vi "d(f2+g2u)_dx4.vi"(1 "x3_":dbl, 4 "x4_":dbl) -> (21 "d(f2+g2u)/dx4":dbl)   [LabVIEW 2014]
uses:
  <vilib>/Simulation/Implementation/Shared/SIMSCR Execution Mode.ctl
  <vilib>/Simulation/Scripting/Companion Diagram/SimConfigNode/SimParams.ctl
  <vilib>/Simulation/Scripting/Companion Diagram/SimConfigNode/_simSolvers.ctl
  <vilib>/Simulation/Param Hierarchy/Typedefs/SIMPH Param Control Actions.ctl
  <vilib>/Simulation/Implementation/Shared/NILVSim_ParamChanged.vi
  <vilib>/Simulation/Implementation/Shared/NILVSIM_BeginStep.vi
  <vilib>/Simulation/Implementation/Shared/NILVSim_Manager.vi
  <vilib>/Utility/error.llb/Clear Errors.vi
  <vilib>/Simulation/Implementation/Shared/NILVSim_FinalizeModel.vi
  <vilib>/Simulation/Implementation/Shared/SIM Unbundle Sim Info.vi
  <vilib>/Simulation/Implementation/Shared/SIMSH Read Queue.vi
  <vilib>/Simulation/Implementation/Shared/NILVSim_Initialize.vi
  <vilib>/Simulation/Utility/Implementation/NILVSim Get Time and IsAcceptedStep.vi
  <vilib>/Simulation/Implementation/Shared/NILVSim_GetModelError.vi
  <vilib>/Simulation/Implementation/Shared/SIM SimErrorHandler.vi
  <vilib>/Simulation/Implementation/Shared/SIM Bundle Sim Info.vi
  <vilib>/Simulation/Scripting/Companion Diagram/SimConfigNode/SimDog.xnode
  <vilib>/Simulation/Implementation/XNodeFramework/SimXNode/SimX.xnode
  <vilib>/Simulation/Implementation/Shared/NI_SIM_Implementation.lvlib
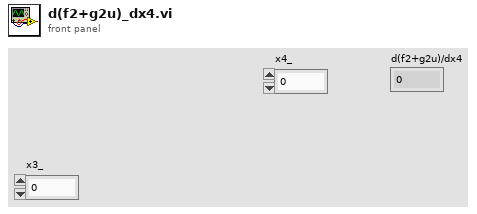
[diagram p1: front panel]
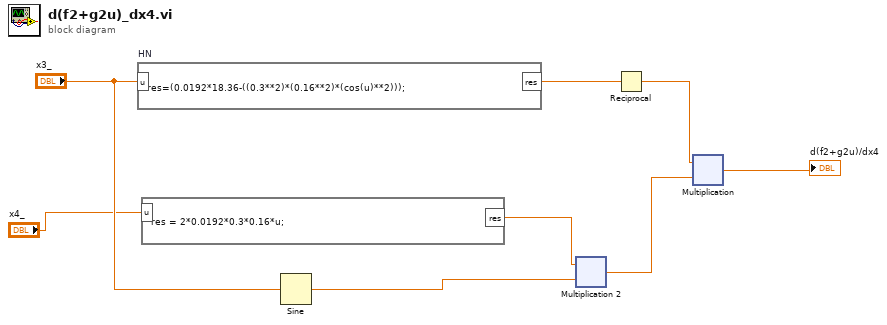
[diagram p0: block diagram]
diagram:
  n1 = formula code="res=(0.0192*18.36-((0.3**2)*(0.16**2)*(cos(u)**2)));" "HN"("u"="x3_") -> ("res"=w8:dbl)
  n2 = formula code="res = 2*0.0192*0.3*0.16*u;" ("Formelknoten")("u"="x4_") -> ("res"=w4:dbl)
  n3 = Sine ("Sinus")(x="x3_") -> (sin(x)=w7:dbl)
  n4 = xnode ("Multiplication 2")("Operand1"=w4, "Operand2"=w7) -> ("Result"=w3:dbl)
  n5 = Reciprocal ("Math\\nFunction")(x=w8) -> (1/x=w2:dbl)
  n6 = xnode "Multiplication"("Operand1"=w2, "Operand2"=w3) -> ("Result"=→"d(f2+g2u)/dx4":dbl)
